vi "Set UA Item.vi"(0 "OPC UA server refnum in":T3, 1 "Parent Folder Id In":string, 5 "Item Name In":string, 7 "data type in":T2=12 items=["Boolean"=1, "SByte"=2, "Byte"=3, "Int16"=4, "UInt16"=5, "Int32"=6, "UInt32"=7, "Int64"=8, "UInt64"=9, "Float"=10, "Double"=11, "String"=12, "DateTime"=13, "ByteString"=15, "Array of Boolean"=101, "Array of SByte"=102, "Array of Byte"=103, "Array of Int16"=104, "Array of UInt16"=105, "Array of Int32"=106, "Array of UInt32"=107, "Array of Int64"=108, "Array of UInt64"=109, "Array of Float"=110, "Array of Double"=111, "Array of String"=112, "Array of DateTime"=113, "Array of ByteString"=115, "Matrix of Boolean"=201, "Matrix of SByte"=202, "Matrix of Byte"=203, "Matrix of Int16"=204, "Matrix of UInt16"=205, "Matrix of Int32"=206, "Matrix of UInt32"=207, "Matrix of Int64"=208, "Matrix of UInt64"=209, "Matrix of Float"=210, "Matrix of Double"=211, "Matrix of String "=212, "Matrix of DateTime"=213, "Matrix of ByteString"=215], 9 "access level in":u16(ring)=3 items=["read-only"=1, "write-only"=2, "read/write"=3], 11 "error in (no error)":errorcluster, 12 "Description In  (opt)":string) -> (4 "OPC UA server refnum out":T3, 6 "Item Id Out":string, 8 "OPC UA variable node refnum out":T1, 15 "error out":errorcluster)   [LabVIEW 2024]
uses:
  <vilib>/OPCUA/controls/OPC UA Server Refnum.ctl
  <vilib>/OPCUA/controls/Data Type.ctl
  <vilib>/OPCUA/controls/OPC UA Variable Node Refnum.ctl
  <vilib>/OPCUA/NI OPC UA Server.lvlib
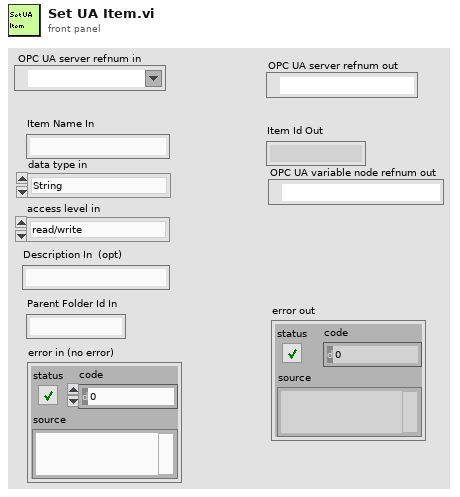
[diagram p1: front panel]
types:
  T1 = typedef "OPC UA Variable Node Refnum.ctl" = refnum<k21>
  T2 = typedef "Data Type.ctl" = u16
  T3 = typedef "OPC UA Server Refnum.ctl" = refnum<k21>
  T4 = cluster{"name":string, "data type":T2, "access level":u16, "description":string}
  T5 = typedef "NodeId.ctl" = string
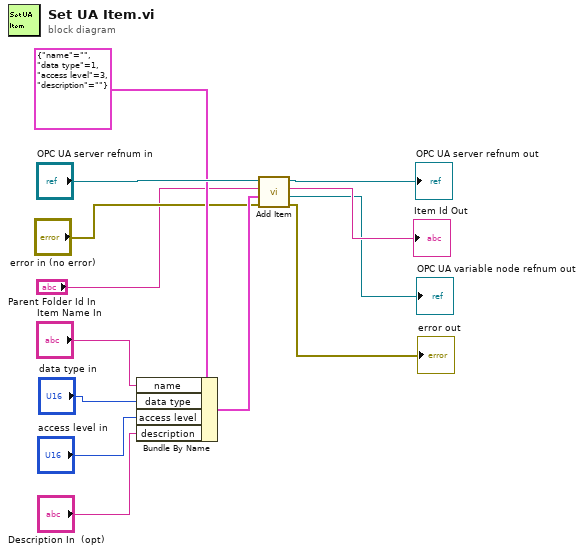
[diagram p0: block diagram]
diagram:
  n1 = Bundle By Name(cluster=T4 {"name"="", "data type"=1, "access level"=3, "description"=""} ("item"), "name"="Item Name In", "data type"="data type in", "access level"="access level in", "description"="Description In  (opt)") -> (w6:T4)
  n2 = call <vilib>:"Add Item.vi"("error in (no error)"="error in (no error)", "item"=w6, "parent folder node ID"="Parent Folder Id In", "OPC UA server refnum in"="OPC UA server refnum in") -> ("error out"=→"error out":errorcluster, "OPC UA variable node refnum out"=→"OPC UA variable node refnum out":T1, "item node ID"=→"Item Id Out":T5, "OPC UA server refnum out"=→"OPC UA server refnum out":T3)  [unwired: 3 in]
